vi "CPP_Aeroprobe.vi"() -> (5 "Plug in titles":string[](array[string]), 7 "Plug in values":string[](array[string]))   [LabVIEW 2016]
uses:
  Controls/AeroprobeType.ctl
  Controls/AeroprobeOrientation.ctl
  ADAM Client/Sub VIs/ADAM Controls/Ch_description_ADAM.ctl
  ADAM Client/Sub VIs/ADAM Controls/Module_type_ADAM.ctl
  ADAM Client/Sub VIs/ADAM Controls/Function_ADAM.ctl
  ADAM Client/Sub VIs/ADAM Controls/Channel_State.ctl
  ADAM Client/Sub VIs/ADAM Controls/Calib_type_ADAM.ctl
  ADAM Client/Sub VIs/ADAM Controls/Address.ctl
  Controls/AeroprobeAngle.ctl
  ADAM Client/Sub VIs/ADAM Controls/Update_scan_value.ctl
  <vilib>/Analysis/baseanly.llb/Mean (DBL).vi
  Globals/Constants_global.vi
  Globals/Meas_global.vi
  Globals/Trav_pos_global.vi
  <vilib>/Utility/file.llb/Write Delimited Spreadsheet (DBL).vi
  <vilib>/Analysis/NI_AALBase.lvlib
panel:
  in  "Angle (deg)":T1=30.0
  in  "Probe Orientation":T2=90 items=["Horizontal"=0, "Diagonal"=45, "Vertical"=90, "User Defined"=999]
  in  "Probe Type":T3=12 items=["5-Hole Probe"=5, "OmniProbe"=12]
  out "MDZeroesVars":string[](array[string])
  out "MDZeroesMeans":string[](array[string])
  out "AeroFlow Output":cluster{string, string}[](array[cluster]) caption="Plug In Titles                                   Plug In Values"
  out "ZeroMeans&Vars":dbl[](array[numeric])
  out "ADAM Chs":T4[](array[typedef]) {"Duty" format="%016b"; "D" format="%#_5g"; "C" format="%#_5g"; "B" format="%#_5g"; "A" format="%#_5g"}
  in  "SaveTimeSeries?":bool
  in  "Mode":enum32{"Measure", "Take Zeroes"}(radio)
  in  "RunManually?":bool
  in  "MeanOrFull":bool
  in  "Graphs":bool
  in  "Downsampler":i32=20
  in  "Calibration Folder Path":path
  in  "Correction File Path":path
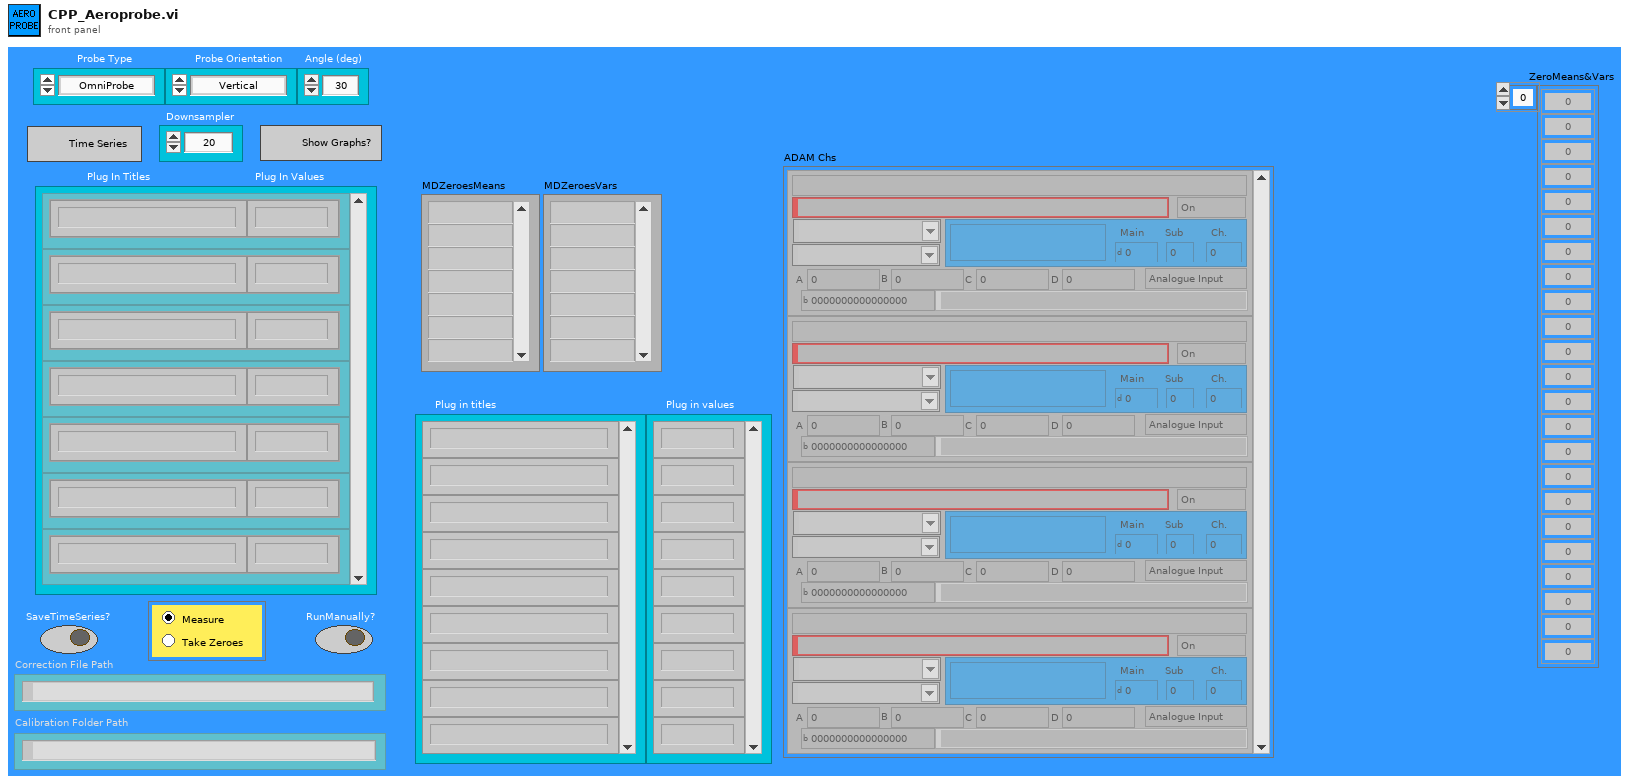
[diagram p1: front panel]
types:
  T1 = typedef "AeroprobeAngle.ctl" = dbl
  T2 = typedef "AeroprobeOrientation.ctl" = u16
  T3 = typedef "AeroprobeType.ctl" = u16
  T4 = typedef "Ch_description_ADAM.ctl" = cluster{"Ch Name":string, "Type":T5, "Function":T6, "Ch State":T7, "Calibration type":T8, "A":dbl, "B":dbl, "C":dbl, "D":dbl, "Comments":string, "Address":T9, "String":string, "Duty":u16}
  T5 = typedef "Module_type_ADAM.ctl" = string
  T6 = typedef "Function_ADAM.ctl" = enum16{"Analogue Input", "Digital Input", "Event counter", "Event rate", "Analogue Output", "Digital Output", "Relay Output"}
  T7 = typedef "Channel_State.ctl" = enum16{"On", "Off", "Always On", "Always Off"}
  T8 = typedef "Calib_type_ADAM.ctl" = string
  T9 = typedef "Address.ctl" = cluster{"Main":i32, "Ch.":i32, "Sub":i32, "Port Name":string}
  T10 = enum16{"Raw Ends", "Mean Ends", "NaNd Ends", "Zeroed Ends"}
  T11 = enum16{"Save no data", "Save data in new files", "Save data in existing files"}
  T12 = typedef "Post_Process.ctl" = enum16{"Take New Data", "Post Process Raw Data File"}
  T13 = typedef "Analysis_info_cluster.ctl" = cluster{"Colour":u32, "Inst type":T14, "Inst name":string, "Symbol":string, "Code name":string, "Extra Info":string, "Inst Array":T15, "Extra Titles":string[], "Extra Values":string[], "U":dbl, "u^2":dbl, "u^3":dbl, "u^4":dbl, "Skew_u":dbl, "Kurt_u":dbl, "Sd Error in Mean":dbl, "% u'/U":dbl, "X":dbl, "Y":dbl, "Z":dbl, "Timescale integral Estimate":dbl, "Sd Error in Variance":dbl, "Calib File":path, "Calib Constants":dbl[], "Output Position":bool, "Full Stats":bool, "Av Sampling Rate":dbl, "Av No of Samples":dbl, "Total Meas Time (s)":dbl, "ADAM Ch Name":string, "Max value":dbl, "Min value":dbl}
  T14 = typedef "Inst_type.ctl" = enum16{"Propeller anemometer", "Raw voltage", "Pressure Transducer", "Pitot-static tube", "Preston tube", "Hot wire", "Cross wire 1", "Cross wire 2", "Generic Linear", "Generic Polynomial", "Generic BackPoly", "Fast FID", "Thermocouple", "Cold wire", "Pulsed Wire", "LDA Vel", "LDA Tran time", "LDA Arr time", "Microphone"}
  T15 = typedef "Instrument_Array.ctl" = enum16{"PWA", "LDA", "Analogue"}
  T16 = typedef "Traverse_cluster.ctl" = cluster{"Start X":sgl, "Start Y":sgl, "Start Z":sgl, "End X":sgl, "End Y":sgl, "End Z":sgl, "No. of pts.":i32, "Spacing":T17, "Filename":path, "Tunnel Speed":dbl, "Averaging time (min)":dbl, "Extra Commands":string, "Carrier_1 Q (l/min)":dbl, "Carrier_2 Q (l/min)":dbl, "Trace Gas Concentration (%)":dbl, "Specific Arguments":string, "Comments":string, "Row No":i32, "Row Type Selector":T18, "Completion time":string, "Row Duration (mins)":dbl, "No. of Valid pts.":i32, "Meas Setup File":string}
  T17 = typedef "Spacing.ctl" = enum16{"Linear", "Log", "Gauss", "Specified", "N/A"}
  T18 = typedef "Multi_run_mode.ctl" = enum16{"Move Traverse Only", "Set Tunnel Speed Only", "Set Source Only", "Set Measurement Conditions", "Single Measurement", "Vertical Profile", "Lateral Profile", "Longitudinal Profile", "Explore Volume", "Multi-Axis Profile", "Auto Calibrate", "Meas Fast FID Bkgnd", "Check Beam Power", "Scanning Valve Measurement", "Run VI Named:", "Set ADAM Ch", "Wait (minutes)", "Send Message", "Synchronize With:", "Fall Back to this Row", "Turn Off Row Repeating", "Blank Row", "Traverse 3D Volume"}
  T19 = typedef "Update_scan_value.ctl" = cluster{"Channel Name":string, "New Value":dbl}
  T20 = typedef "Time_Trace_Cluster.ctl" = cluster{"Weighting":dbl[], "Time (s)":dbl[], "Voltage":dbl[], "Eng Values":dbl[]}
  T21 = cluster{"CleanVmagUVWCone":dbl[][], "CleanXvals":i32[]}
  T22 = typedef "SanityCluster.ctl" = cluster{"PressureErrors":bool[][], "Plug in titles":string[]}
  T23 = cluster{"   Vmag          U               V              W        Cone":dbl[][], "Xvals":i32[]}
  T24 = cluster{"element":string, "RingText.Text":string}
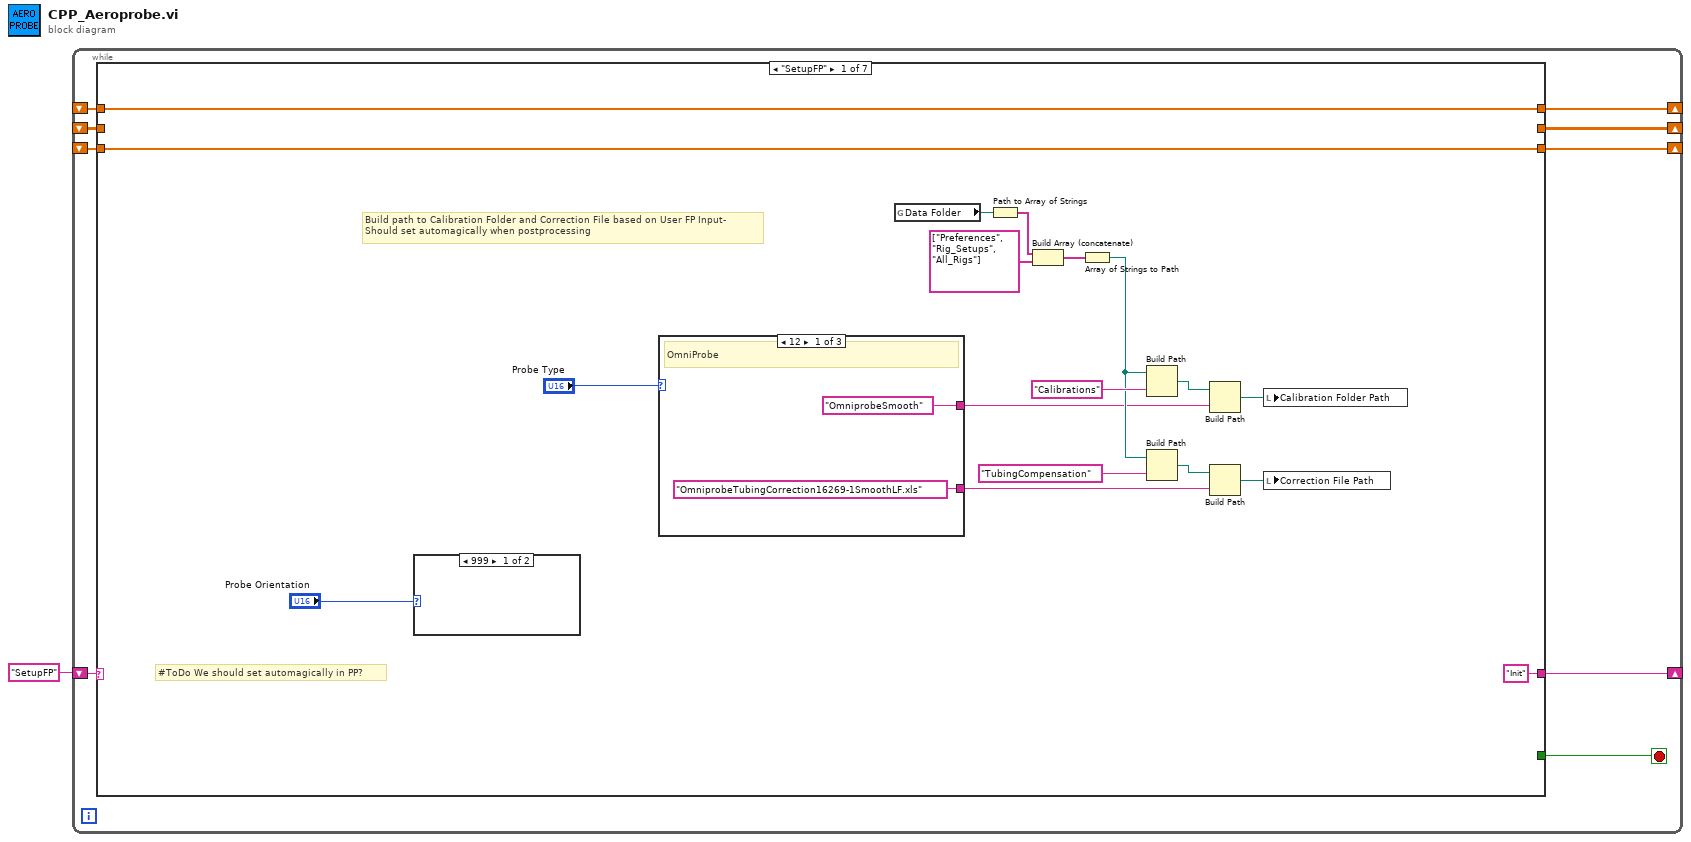
[diagram p0: block diagram]
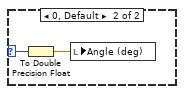
[diagram p2: hidden frame]
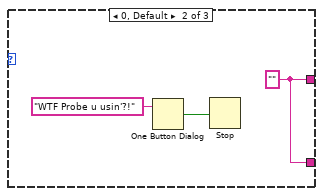
[diagram p3: hidden frame]
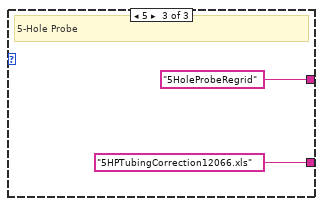
[diagram p4: hidden frame]
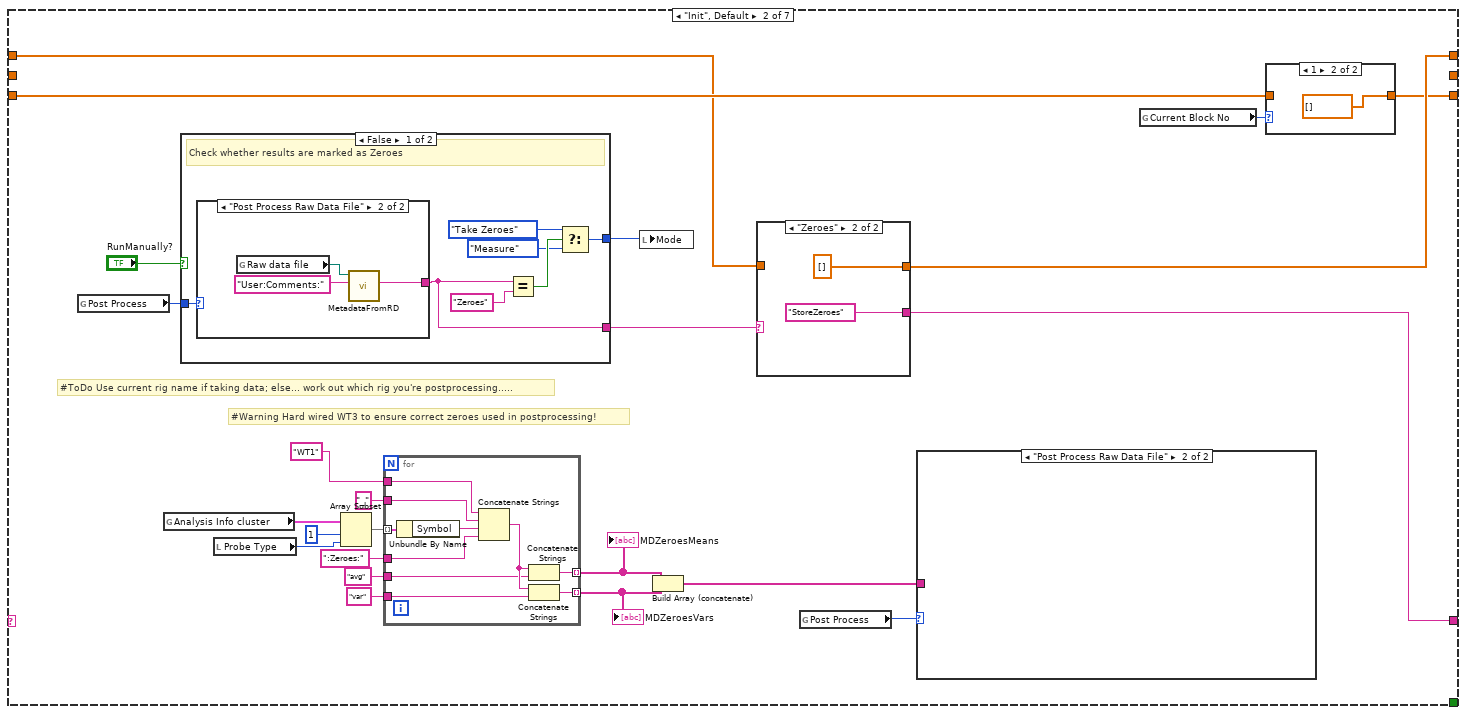
[diagram p5: hidden frame]
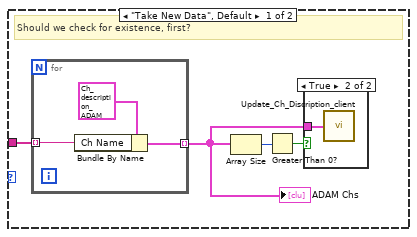
[diagram p6: hidden frame]
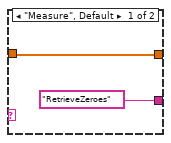
[diagram p8: hidden frame]
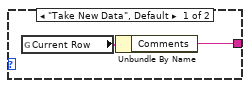
[diagram p9: hidden frame]
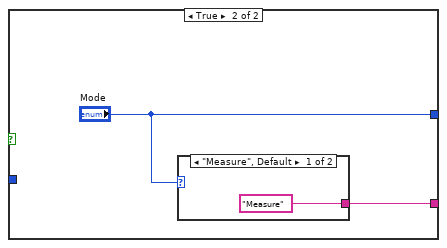
[diagram p10: hidden frame]
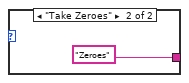
[diagram p11: hidden frame]
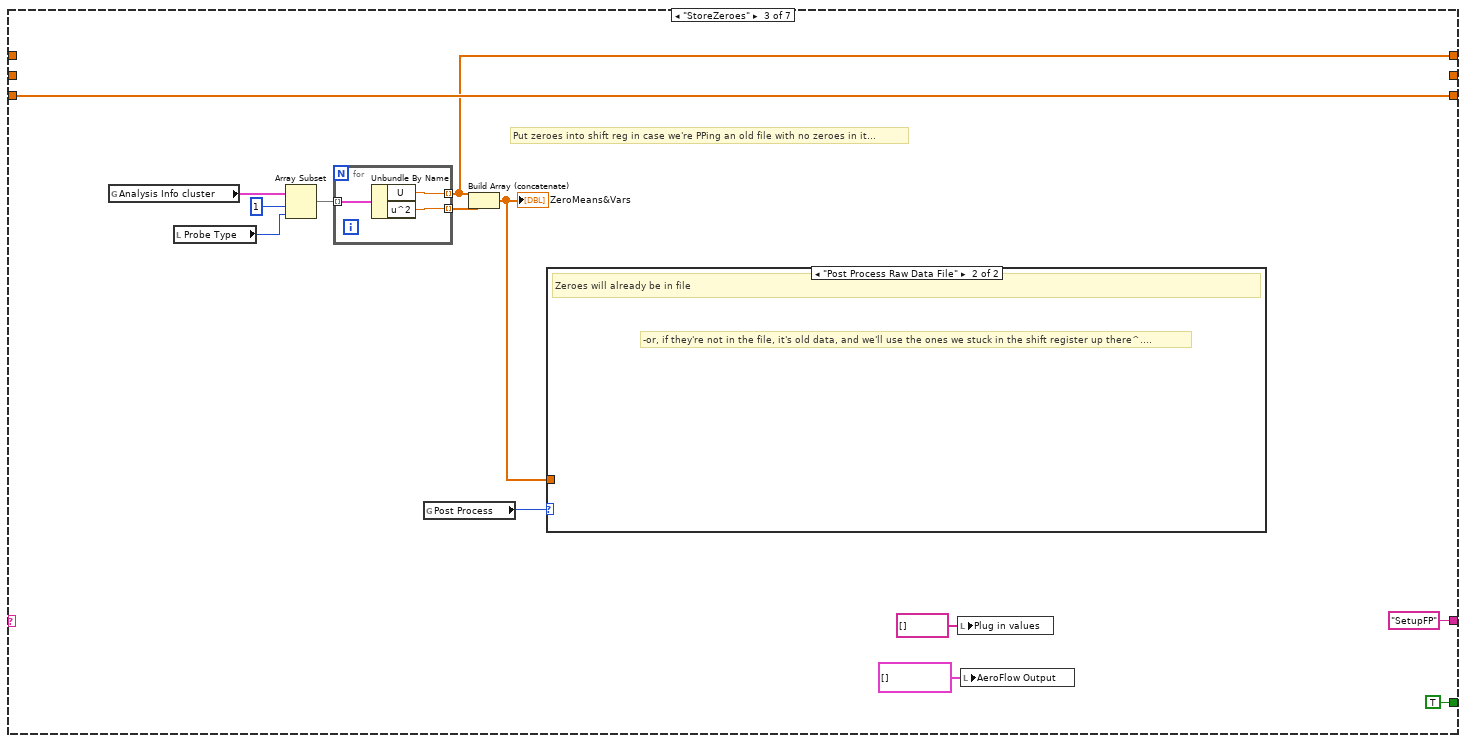
[diagram p13: hidden frame]
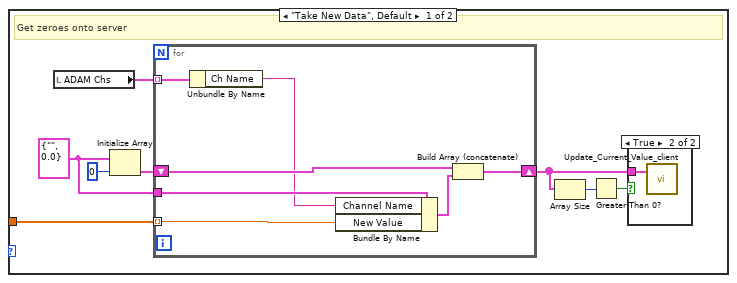
[diagram p14: hidden frame]
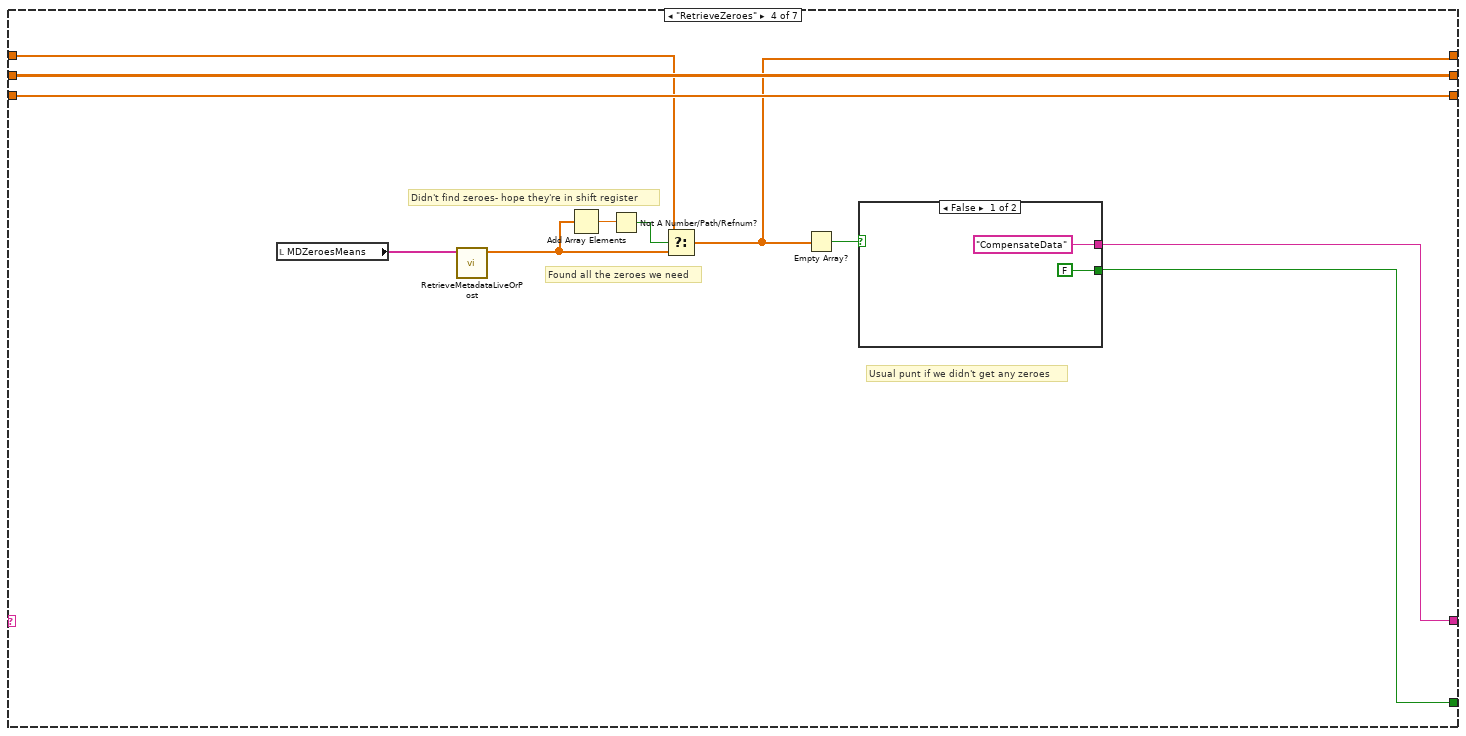
[diagram p16: hidden frame]
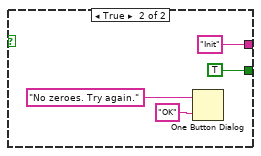
[diagram p17: hidden frame]
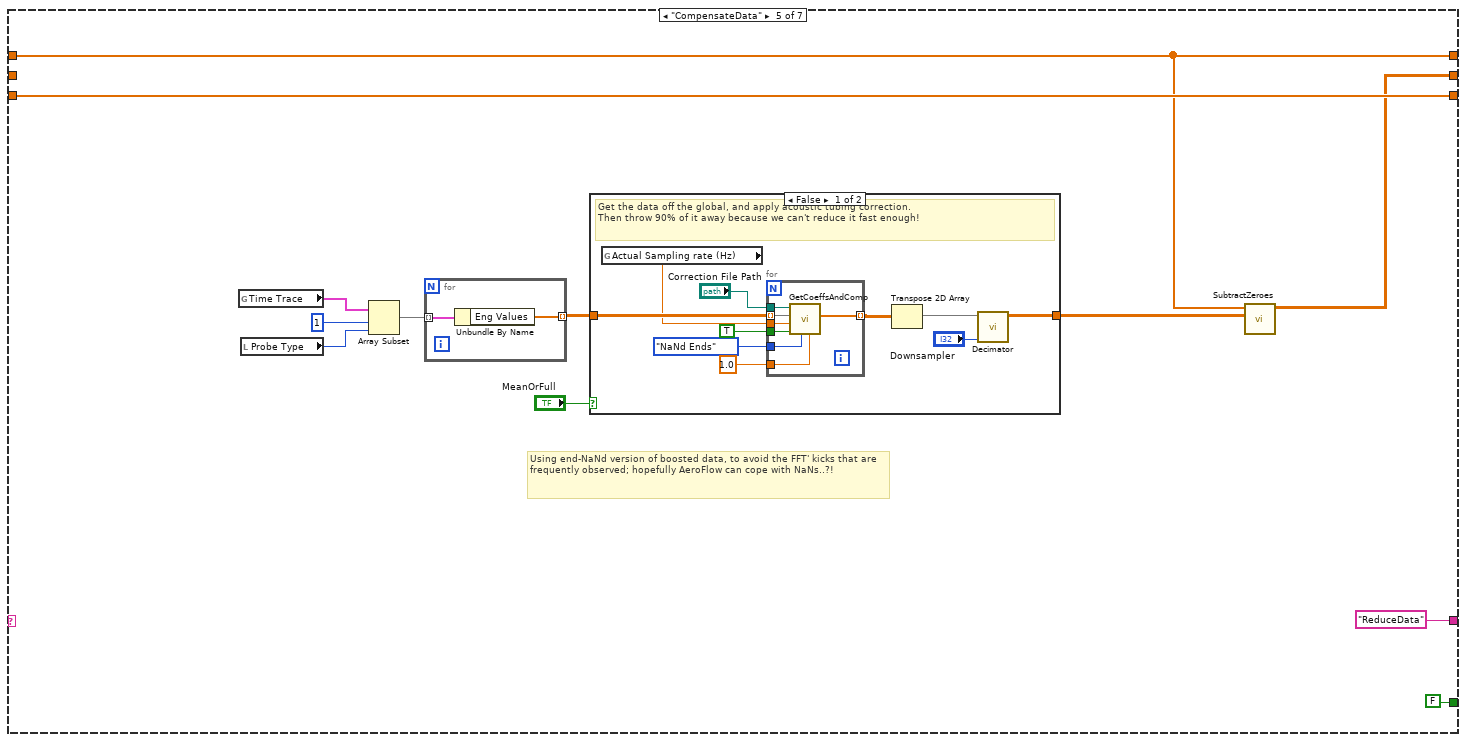
[diagram p18: hidden frame]
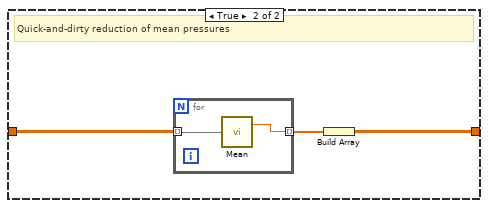
[diagram p19: hidden frame]
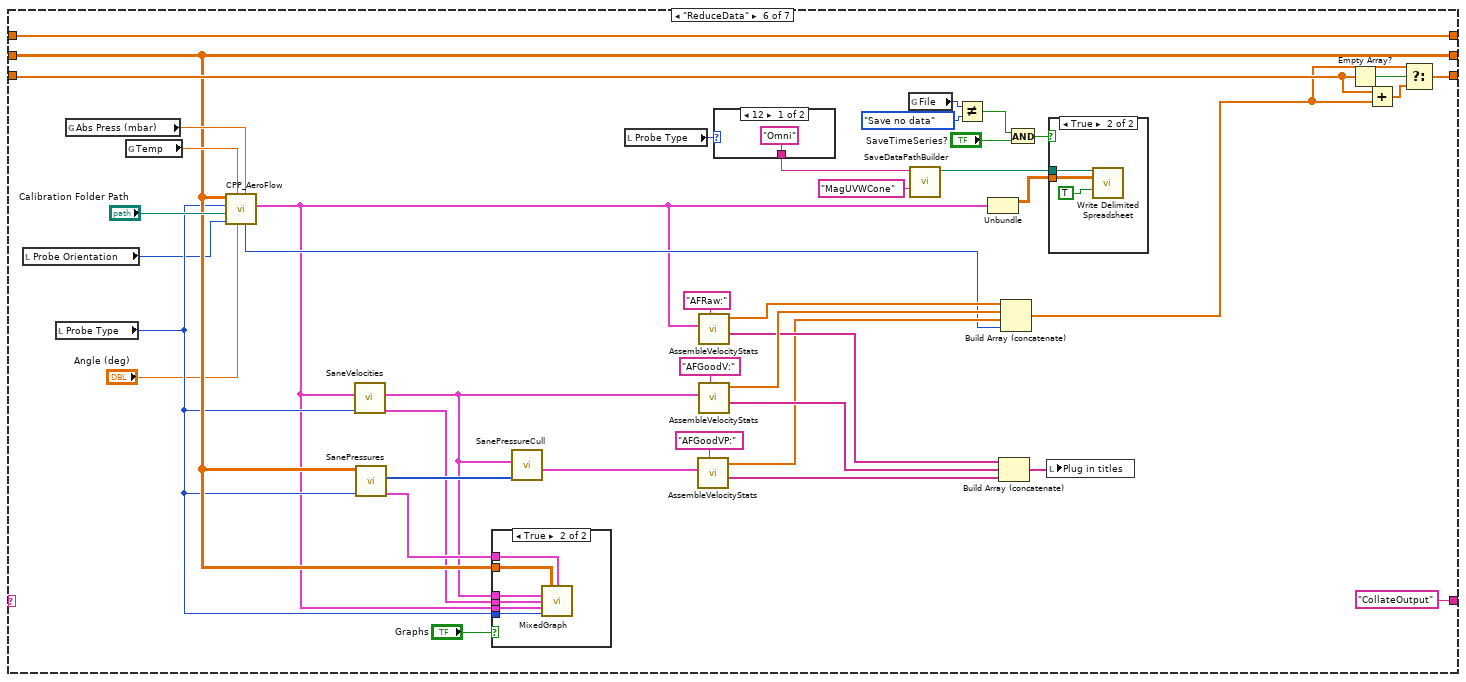
[diagram p20: hidden frame]
diagram:
  n1 = while {
    shift-right: [w9] -> _
    shift-left: "SetupFP" -> [w10]
    shift-right: [w8] -> _
    shift-left: _ -> [w7]
    shift-right: [w6] -> _
    shift-left: _ -> [w5]
    shift-right: [w3] -> _
    shift-left: _ -> [w2]
    stop <- w4 stop-if-true
    n2 = case shown="\"SetupFP\"" w10 {
      tunnel: ["Init" w43 "SetupFP" w138 "ReduceData" "CollateOutput" "Init"] -> w9
      tunnel: [w28 w60 w107 w133 w159 w226 w276] -> w8
      tunnel: w7 -> [w28 w44 _ w135 w159 w226 w276]
      tunnel: [w27 w59 w113 w143 w161 w222 w270] -> w6
      tunnel: w5 -> [w27 w58 w113 w143 w161 w225 w270]
      tunnel: [_ _ TRUE w137 FALSE _ TRUE] -> w4
      tunnel: [_ _ _ w142 w156 w198 w272] -> w3
      tunnel: w2 -> [_ _ _ w142 _ w198 w272]
      frame "SetupFP" {
        # "#ToDo We should set automagically in PP?"
        # "Build path to Calibration Folder and Correction File based on User FP Input-\nShould set automagically when postprocessing"
        n3 = case shown="999" "Probe Orientation" {
          selector: "Probe Orientation" -> [_ w30]
          frame 999 {
          }
          frame 0, Default {
            n4 = To Double Precision Float(number=w30) -> (double precision float=w29:dbl)
            n5 = local write "Angle (deg)"(w29) -> ()
          }
        }
        n6 = case shown="12" "Probe Type" {
          tunnel: ["OmniprobeTubingCorrection16269-1SmoothLF.xls" ("Tubing Compensation File") w35 "5HPTubingCorrection12066.xls" ("Tubing Compensation File")] -> w18
          tunnel: ["OmniprobeSmooth" ("Calibration Folder") w35 "5HoleProbeRegrid" ("Calibration Folder")] -> w17
          frame 12 {
            # "OmniProbe"
          }
          frame 0, Default {
            w35 = "" ("Calibration Folder")
            n7 = One Button Dialog(message="WTF Probe u usin'?!") -> (true=w33:bool)  [unwired: 1 in]
            n8 = Stop(stop? (T)=w33) -> ()
          }
          frame 5 {
            # "5-Hole Probe"
          }
        }
        n9 = global read "Constants_global.vi" "Data Folder"() -> (w22:path)
        n10 = Path to Array of Strings(0:w22) -> (2:w25:string[])  [unwired: 1 out]
        n11 = Build Array (concatenate)(w25, string[] ["Preferences", "Rig_Setups", "All_Rigs"] ("array of strings 3")) -> (w23:string[])
        n12 = Array of Strings to Path(0:w23) -> (2:w19:path)  [unwired: 1 in]
        n13 = Build Path(base path=w19, name or relative path="Calibrations") -> (appended path=w15:path)
        n14 = Build Path(base path=w19, name or relative path="TubingCompensation") -> (appended path=w16:path)
        n15 = Build Path(base path=w15, name or relative path=w17) -> (appended path=w14:path)
        n16 = Build Path(base path=w16, name or relative path=w18) -> (appended path=w13:path)
        n17 = local write "Calibration Folder Path"(w14) -> ()
        n18 = local write "Correction File Path"(w13) -> ()
      }
      frame "Init", Default {
        # "#ToDo Use current rig name if taking data; else... work out which rig you're postprocessing....."
        # "#Warning Hard wired WT3 to ensure correct zeroes used in postprocessing!"
        n19 = global read "Meas_global.vi" "Post Process"() -> (w54:T12)
        n20 = global read "Meas_global.vi" "Analysis Info cluster"() -> (w52:T13[])
        n21 = case shown="False" "RunManually?" {
          tunnel: [w89 "Mode"] -> w55
          tunnel: w54 -> [w84 _]
          tunnel: [w83 w95] -> w45
          frame False {
            # "Check whether results are marked as Zeroes"
            n22 = case shown="\"Post Process Raw Data File\"" w84 {
              tunnel: [w90 w92] -> w83
              frame "Take New Data", Default {
                n23 = global read "Trav_pos_global.vi" "Current Row"() -> (w91:T16)
                n24 = Unbundle By Name(w91) -> ("Comments"=w90:string)
              }
              frame "Post Process Raw Data File" {
                n25 = global read "Meas_global.vi" "Raw data file"() -> (w94:path)
                n26 = call "MetadataFromRD.vi"("ChannelName"="User:Comments:", "Raw data file"=w94) -> ("ValueString"=w92:string)  [unwired: 8 in, 1 out]
              }
            }
            n27 = Equal?(x=w83, y="Zeroes") -> (x = y?=w87:bool)
            n28 = Select(t=enum32{"Measure", "Take Zeroes"}."Take Zeroes" ("Mode"), s=w87, f=enum32{"Measure", "Take Zeroes"}."Measure" ("Mode")) -> (s? t:f=w89:enum32{"Measure", "Take Zeroes"})
          }
          frame True {
            n29 = case shown="\"Measure\", Default" "Mode" {
              tunnel: ["Measure" ("y") "Zeroes" ("y")] -> w95
              frame "Measure", Default {
              }
              frame "Take Zeroes" {
              }
            }
          }
        }
        n30 = local read "Probe Type"() -> (w46:T3)
        n31 = Array Subset(array=w52, index=1, length=w46) -> (w51:T13[])
        n32 = for {
          tunnel: w51 -> [w82] mode=indexing
          tunnel: ":Zeroes:" -> [w80]
          tunnel: "avg" -> [w77]
          tunnel: "var" -> [w79]
          tunnel: "_" -> [w76]
          tunnel: "WT1" -> [w75]
          tunnel: [w74] -> w41 mode=indexing
          tunnel: [w73] -> w40 mode=indexing
          n33 = Unbundle By Name(w82) -> ("Symbol"=w81:string)
          n34 = Concatenate Strings(w75, w76, w81, w80) -> (w78:string)
          n35 = Concatenate Strings(w78, w77) -> (w74:string)
          n36 = Concatenate Strings(w78, w79) -> (w73:string)
        }
        "MDZeroesMeans" <- w41
        "MDZeroesVars" <- w40
        n37 = local write "Mode"(w55) -> ()
        n38 = Build Array (concatenate)(w41, w40) -> (w39:string[])
        n39 = case shown="\"Zeroes\"" w45 {
          tunnel: [w70 dbl[] [] ("t")] -> w60
          tunnel: w44 -> [w70 _]
          tunnel: ["RetrieveZeroes" "StoreZeroes"] -> w43
          frame "Measure", Default {
          }
          frame "Zeroes" {
          }
        }
        n40 = global read "Meas_global.vi" "Post Process"() -> (w42:T12)
        n41 = case shown="\"Post Process Raw Data File\"" w42 {
          tunnel: w39 -> [w64 _]
          frame "Take New Data", Default {
            # "Should we check for existence, first?"
            n42 = for {
              tunnel: w64 -> [w67] mode=indexing
              tunnel: [w66] -> w61 mode=indexing
              n43 = Bundle By Name(cluster=T4 {"Ch Name"="", "Type"="Hold Value", "Function"=enum."Analogue Input", "Ch State"=enum."On", "Calibration type"="", "A"=0.0, "B"=0.0, "C"=0.0, "D"=0.0, "Comments"="", "Address"={"Main"=0, "Ch."=0, "Sub"=0, "Port Name"=""}, "String"="", "Duty"=0} ("Ch Discription"), "Ch Name"=w67) -> (w66:T4)
            }
            "ADAM Chs" <- w61
            n44 = Array Size(array=w61) -> (size(s)=w63:i32)
            n45 = Greater Than 0?(x=w63) -> (x > 0?=w62:bool)
            n46 = case shown="True" w62 {
              tunnel: w61 -> [_ w65]
              frame False {
              }
              frame True {
                n47 = call "Update_Ch_Discription_client.vi"("Channels to update In"=w65) -> ()  [unwired: 1 out]
              }
            }
          }
          frame "Post Process Raw Data File" {
          }
        }
        n48 = global read "Meas_global.vi" "Current Block No"() -> (w57:i32)
        n49 = case shown="1" w57 {
          tunnel: [w99 dbl[] [] ("t")] -> w59
          tunnel: w58 -> [w99 _]
          frame 0, Default {
          }
          frame 1 {
          }
        }
      }
      frame "StoreZeroes" {
        # "Put zeroes into shift reg in case we're PPing an old file with no zeroes in it..."
        n50 = global read "Meas_global.vi" "Analysis Info cluster"() -> (w111:T13[])
        n51 = local read "Probe Type"() -> (w109:T3)
        n52 = Array Subset(array=w111, index=1, length=w109) -> (w110:T13[])
        n53 = for {
          tunnel: w110 -> [w132] mode=indexing
          tunnel: [w131] -> w107 mode=indexing
          tunnel: [w130] -> w108 mode=indexing
          n54 = Unbundle By Name(w132) -> ("U"=w131:dbl, "u^2"=w130:dbl)
        }
        n55 = global read "Meas_global.vi" "Post Process"() -> (w105:T12)
        n56 = Build Array (concatenate)(w107, w108) -> (w106:dbl[])
        "ZeroMeans&Vars" <- w106
        n57 = case shown="\"Post Process Raw Data File\"" w105 {
          tunnel: w106 -> [w114 _]
          frame "Take New Data", Default {
            w116 = T19 {"Channel Name"="", "New Value"=0.0} ("Update Scan Value Cluster")
            # "Get zeroes onto server"
            n58 = local read "ADAM Chs"() -> (w115:T4[])
            n59 = Initialize Array(w116, 0 ("Dimension Size")) -> (w120:T19[])
            n60 = for {
              shift-right: [w129] -> w117
              shift-left: w120 -> [w128]
              tunnel: w114 -> [w126] mode=indexing
              tunnel: w115 -> [w125] mode=indexing
              tunnel: w116 -> [w127]
              n61 = Unbundle By Name(w125) -> ("Ch Name"=w124:string)
              n62 = Bundle By Name(cluster=w127, "Channel Name"=w124, "New Value"=w126) -> (w123:T19)
              n63 = Build Array (concatenate)(w128, w123) -> (w129:T19[])
            }
            n64 = Array Size(array=w117) -> (size(s)=w118:i32)
            n65 = Greater Than 0?(x=w118) -> (x > 0?=w119:bool)
            n66 = case shown="True" w119 {
              tunnel: w117 -> [_ w122]
              frame False {
              }
              frame True {
                n67 = call "Update_Current_Value_client.vi"("Update array in"=w122) -> ()  [unwired: 1 in]
              }
            }
          }
          frame "Post Process Raw Data File" {
            # "-or, if they're not in the file, it's old data, and we'll use the ones we stuck in the shift register up there^...."
            # "Zeroes will already be in file"
          }
        }
        n68 = local write "Plug in values"(string[] [] ("Plug in values")) -> ()
        n69 = local write "AeroFlow Output"(cluster{string, string}[] [] ("AeroFlow Output")) -> ()
      }
      frame "RetrieveZeroes" {
        # "Didn't find zeroes- hope they're in shift register"
        # "Found all the zeroes we need"
        # "Usual punt if we didn't get any zeroes"
        n70 = local read "MDZeroesMeans"() -> (w141:string[])
        n71 = call "RetrieveMetadataLiveOrPost.vi"("ChannelsToGet"=w141) -> ("ChannelValues"=w134:dbl[])  [unwired: 10 in]
        n72 = Add Array Elements(numeric array=w134) -> (sum=w140:dbl)
        n73 = Not A Number/Path/Refnum?(number/path/refnum=w140) -> (NaN/Path/Refnum?=w136:bool)
        n74 = Select(t=w135, s=w136, f=w134) -> (s? t:f=w133:dbl[])
        n75 = Empty Array?(array=w133) -> (empty?=w139:bool)
        n76 = case shown="False" w139 {
          tunnel: ["CompensateData" "Init"] -> w138
          tunnel: [FALSE TRUE] -> w137
          frame False {
          }
          frame True {
            n77 = One Button Dialog(message="No zeroes. Try again.", button name ("OK")="OK") -> ()  [unwired: 1 out]
          }
        }
      }
      frame "CompensateData" {
        # "Using end-NaNd version of boosted data, to avoid the FFT' kicks that are frequently observed; hopefully AeroFlow can cope with NaNs..?!"
        n78 = global read "Meas_global.vi" "Time Trace"() -> (w154:T20[])
        n79 = local read "Probe Type"() -> (w150:T3)
        n80 = Array Subset(array=w154, index=1, length=w150) -> (w152:T20[])
        n81 = for {
          tunnel: w152 -> [w163] mode=indexing
          tunnel: [w162] -> w151 mode=indexing
          n82 = Unbundle By Name(w163) -> ("Eng Values"=w162:dbl[])
        }
        n83 = case shown="False" "MeanOrFull" {
          tunnel: [w168 w183] -> w160
          tunnel: w151 -> [w167 w182]
          frame False {
            # "Get the data off the global, and apply acoustic tubing correction. \nThen throw 90% of it away because we can't reduce it fast enough!"
            n84 = global read "Meas_global.vi" "Actual Sampling rate (Hz)"() -> (w166:dbl)
            n85 = for {
              tunnel: w167 -> [w180] mode=indexing
              tunnel: [w176] -> w171 mode=indexing
              tunnel: TRUE ("Apply Phase Correction?") -> [w179]
              tunnel: "Correction File Path" -> [w178]
              tunnel: w166 -> [w177]
              tunnel: T10."NaNd Ends" ("EndTreatment") -> [w175]
              tunnel: 1.0 ("EndTrimLength(%)") -> [w174]
              n86 = call "GetCoeffsAndComp.vi"("EndTrimLength(%)"=w174, "EndTreatment"=w175, "Apply Phase Correction?"=w179, "Actual Sampling rate (Hz)"=w177, "mutedData"=w180, "TubingCorrectionFile"=w178) -> ("boostedData"=w176:dbl[])  [unwired: 5 in]
            }
            n87 = Transpose 2D Array(2D array=w171) -> (transposed array=w170:dbl[][])
            n88 = call "Decimator.vi"("Decimator"="Downsampler", "Array In"=w170) -> ("DecimatedArrayOut"=w168:dbl[][])  [unwired: 9 in]
          }
          frame True {
            # "Quick-and-dirty reduction of mean pressures"
            n89 = for {
              tunnel: w182 -> [w185] mode=indexing
              tunnel: [w184] -> w181 mode=indexing
              n90 = call-poly <vilib>:"Mean.vi"("X"=w185) -> ("mean"=w184:dbl)  [unwired: 1 out]
            }
            n91 = Build Array(w181) -> (w183:dbl[][])
          }
        }
        n92 = call "SubtractZeroes.vi"("RawPressure"=w160, "Zeroes"=w159) -> ("ZeroedPressure"=w156:dbl[][])  [unwired: 9 in]
      }
      frame "ReduceData" {
        n93 = local read "Probe Orientation"() -> (w186:T2)
        n94 = local read "Probe Type"() -> (w192:T3)
        n95 = global read "Meas_global.vi" "Abs Press (mbar)"() -> (w220:dbl)
        n96 = global read "Meas_global.vi" "Temp"() -> (w219:dbl)
        n97 = call "CPP_AeroFlow.vi"("Pressure (mBar)"=w220, "Probe Angle (deg)"="Angle (deg)", "Temperature (C)"=w219, "Probe Orientation"=w186, "Calibration Folder Path"="Calibration Folder Path", "Probe Type"=w192, "ZeroedPressures (mmH2O)"=w198) -> ("Output"=w191:T21, "Time(ms)"=w197:u32)  [unwired: 1 in, 2 out]
        n98 = call "SaneVelocities.vi"("Probe Type"=w192, "DataIn"=w191) -> ("VelocityErrors"=w190:T22, "DataOut"=w189:T23)  [unwired: 8 in]
        n99 = call "SanePressures.vi"("Probe Type"=w192, "ZeroedPressures"=w198) -> ("PressureIssues"=w196:T22, "XvalsGoodP"=w195:i32[])  [unwired: 8 in]
        n100 = case shown="True" "Graphs" {
          tunnel: w198 -> [_ w238]
          tunnel: w196 -> [_ w237]
          tunnel: w192 -> [_ w236]
          tunnel: w191 -> [_ w235]
          tunnel: w190 -> [_ w234]
          tunnel: w189 -> [_ w233]
          frame False {
          }
          frame True {
            n101 = call "MixedGraph.vi"("ZeroedPressures"=w238, "PressureSanity"=w237, "DataInClean"=w233, "CleaningErrors"=w234, "DataInRaw"=w235, "Probe Type"=w236) -> ()  [unwired: 10 in]
          }
        }
        n102 = call "SanePressureCull.vi"("GoodPressureXvals"=w195, "DataIn"=w189) -> ("DataOut"=w193:T23)  [unwired: 9 in]
        n103 = local read "Probe Type"() -> (w200:T3)
        n104 = call "AssembleVelocityStats.vi"("TitlePrefix"="AFGoodVP:", "DataIn"=w193) -> ("Plug in titles"=w209:string[], "StatsArray"=w208:dbl[])  [unwired: 8 in]
        n105 = call "AssembleVelocityStats.vi"("TitlePrefix"="AFRaw:", "DataIn"=w191) -> ("Plug in titles"=w212:string[], "StatsArray"=w214:dbl[])  [unwired: 8 in]
        n106 = call "AssembleVelocityStats.vi"("TitlePrefix"="AFGoodV:", "DataIn"=w189) -> ("Plug in titles"=w211:string[], "StatsArray"=w213:dbl[])  [unwired: 8 in]
        n107 = case shown="12" w200 {
          tunnel: ["Omni" ("Inst name") "5HP" ("Inst name")] -> w199
          frame 12 {
          }
          frame 5, Default {
          }
        }
        n108 = global read "Meas_global.vi" "File"() -> (w204:T11)
        n109 = call "SaveDataPathBuilder.vi"("DataTypeSuffix"="MagUVWCone", "Inst name"=w199) -> ("Path name Out"=w206:path)  [unwired: 9 in]
        n110 = Not Equal?(x=w204, y=T11."Save no data" ("File")) -> (x != y?=w201:bool)
        n111 = Unbundle(w191) -> ("CleanVmagUVWCone"=w194:dbl[][])  [unwired: 1 out]
        n112 = Build Array (concatenate)(w212, w211, w209) -> (w188:string[])
        n113 = Build Array (concatenate)(w214, w213, w208, w197) -> (w215:dbl[])
        n114 = And(x=w201, y="SaveTimeSeries?") -> (x .and. y?=w202:bool)
        n115 = local write "Plug in titles"(w188) -> ()
        n116 = case shown="True" w202 {
          tunnel: w194 -> [_ w231]
          tunnel: w206 -> [_ w232]
          frame False {
          }
          frame True {
            n117 = call-poly <vilib>:"Write Delimited Spreadsheet.vi"("file path (dialog if empty)"=w232, "2D data"=w231, "append to file? (new file:F)"=TRUE) -> ()  [unwired: 11 in, 2 out]
          }
        }
        n118 = Empty Array?(array=w225) -> (empty?=w224:bool)
        n119 = Add(x=w225, y=w215) -> (x+y=w223:dbl[])
        n120 = Select(t=w215, s=w224, f=w223) -> (s? t:f=w222:dbl[])
      }
      frame "CollateOutput" {
        # "Calculate ensemble average"
        n121 = global read "Meas_global.vi" "Current Block No"() -> (w273:i32)
        n122 = local read "Downsampler"() -> (w269:i32)
        n123 = local read "MeanOrFull"() -> (w268:bool)
        n124 = local read "Angle (deg)"() -> (w242:T1)
        n125 = local read "Calibration Folder Path"() -> (w258:path)
        n126 = local read "Correction File Path"() -> (w260:path)
        n127 = Divide(x=w270, y=w273) -> (x/y=w271:dbl[])
        n128 = Get Date/Time In Seconds() -> (seconds since 1Jan1904=w265:timestamp)
        n129 = Number To Decimal String(number=w269) -> (decimal integer string=w267:string)  [unwired: 1 in]
        n130 = property on="Probe Type" class="Ring (strict)"() -> ("RingText.Text"=w255:string)  [unwired: 2 in, 2 out]
        n131 = property on="Probe Orientation" class="Ring (strict)"() -> ("RingText.Text"=w254:string)  [unwired: 2 in, 2 out]
        n132 = To Double Precision Float(number=w265) -> (double precision float=w264:dbl)
        n133 = Number To Fractional String(number=w271) -> (F-format string=w261:string[])  [unwired: 3 in]
        n134 = Select(t="0", s=w268, f=w267) -> (s? t:f=w263:string)
        n135 = Number To Fractional String(number=w242, precision (6)=i16 2) -> (F-format string=w240:string)  [unwired: 2 in]
        n136 = Number To Fractional String(number=w264, precision (6)=i16 3) -> (F-format string=w262:string)  [unwired: 2 in]
        n137 = Path To String(path=w260) -> (string=w259:string)
        n138 = Path To String(path=w258) -> (string=w257:string)
        n139 = Build Array (concatenate)(w261, w263, w262, w259, w257, w255, w254, w240) -> (w253:string[])
        "Plug in values" <- w253
        n140 = local read "Plug in titles"() -> (w244:string[])
        n141 = Build Array (concatenate)(w244, "AFReduction:Time:(ms)", "Decimation:n:(0 for means only)" ("element"), "Reduction:Timestamp:(ss1-1-1904)" ("element"), "Tubing:Correction:File" ("element"), "Probe:Cal:File" ("element"), "Probe:Type:" ("element"), "Probe:Orientation:" ("element"), "Probe:Angle:(deg)" ("element")) -> (w243:string[])
        "Plug in titles" <- w243
        n142 = for {
          tunnel: w253 -> [w279] mode=indexing
          tunnel: w243 -> [w278] mode=indexing
          tunnel: [w277] -> w252 mode=indexing
          n143 = Bundle("element"=w278, "RingText.Text"=w279) -> (w277:T24)  [unwired: 1 in]
        }
        "AeroFlow Output" <- w252
      }
    }
  }
